vi "F.L.Y Stick Controller.vi"   [LabVIEW 2019]
uses:
  <vilib>/Rock Robotics/WPI/Joystick/WPI_JoystickDeviceEnum.ctl
  F.L.Y Stick Controller Global.vi
types:
  T1 = typedef "WPI_JoystickDeviceEnum.ctl" = enum16{"USB 0", "USB 1", "USB 2", "USB 3", "USB 4", "USB 5"}
  T2 = typedef "WPI_JoystickDevRef.ctl" = cluster{"Device":T1}
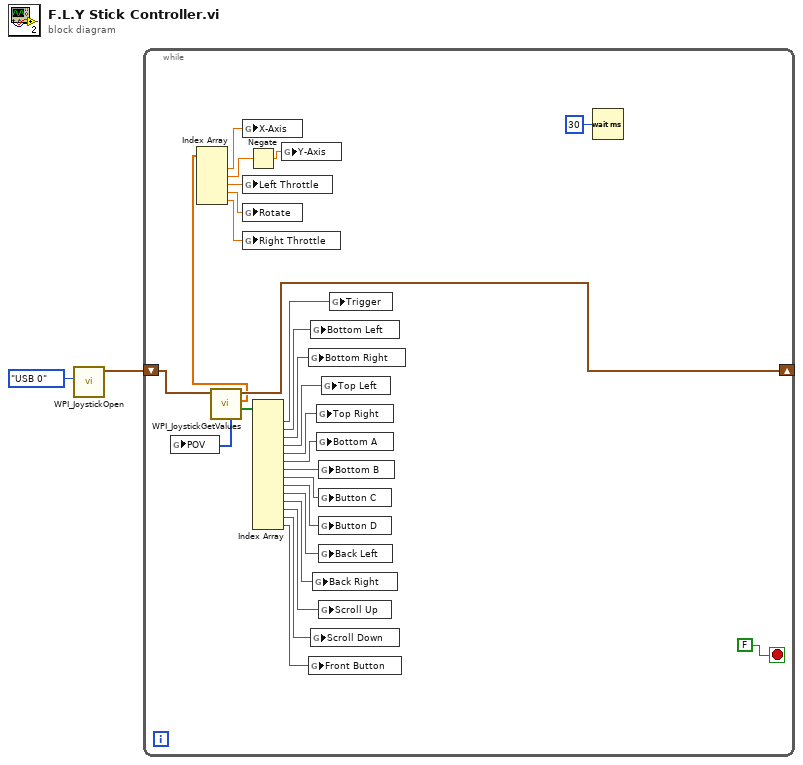
[diagram p0: block diagram]
diagram:
  n1 = call <vilib>:"WPI_JoystickOpen.vi"("JoystickDevice"=WPI_JoystickDeviceEnum."USB 0") -> ("JoystickDevRef"=w2:T2)  [unwired: 10 in]
  n2 = while {
    shift-right: [w27] -> _
    shift-left: w2 -> [w28]
    stop <- FALSE stop-if-true
    n3 = call <vilib>:"WPI_JoystickGetValues.vi"("JoystickDevRef"=w28) -> ("Buttons"=w26:bool[], "Axes"=w11:dbl[], "JoystickDevRef"=w27:T2, "POVs"=w6:i16[])  [unwired: 6 in, 1 out]
    n4 = global write "F.L.Y Stick Controller Global.vi" "POV"(w6) -> ()
    n5 = Index Array(array=w11) -> (element #1=w10:dbl, element #2=w3:dbl, element #3=w9:dbl, element #4=w8:dbl, element #5=w7:dbl)  [unwired: 5 in]
    n6 = global write "F.L.Y Stick Controller Global.vi" "X-Axis"(w10) -> ()
    n7 = global write "F.L.Y Stick Controller Global.vi" "Left Throttle"(w9) -> ()
    n8 = global write "F.L.Y Stick Controller Global.vi" "Rotate"(w8) -> ()
    n9 = global write "F.L.Y Stick Controller Global.vi" "Right Throttle"(w7) -> ()
    n10 = Negate(x=w3) -> (-x=w4:dbl)
    n11 = Index Array(array=w26) -> (element #1=w25:bool, element #2=w24:bool, element #3=w23:bool, element #4=w22:bool, element #5=w21:bool, element #6=w20:bool, element #7=w19:bool, element #8=w18:bool, element #9=w17:bool, element #10=w16:bool, element #11=w15:bool, element #12=w14:bool, element #13=w13:bool, element #14=w12:bool)  [unwired: 14 in]
    n12 = global write "F.L.Y Stick Controller Global.vi" "Y-Axis"(w4) -> ()
    n13 = global write "F.L.Y Stick Controller Global.vi" "Bottom Right"(w23) -> ()
    n14 = global write "F.L.Y Stick Controller Global.vi" "Front Button"(w12) -> ()
    n15 = global write "F.L.Y Stick Controller Global.vi" "Bottom Left"(w24) -> ()
    n16 = global write "F.L.Y Stick Controller Global.vi" "Scroll Down"(w13) -> ()
    n17 = global write "F.L.Y Stick Controller Global.vi" "Back Right"(w15) -> ()
    n18 = global write "F.L.Y Stick Controller Global.vi" "Top Right"(w21) -> ()
    n19 = global write "F.L.Y Stick Controller Global.vi" "Bottom A"(w20) -> ()
    n20 = global write "F.L.Y Stick Controller Global.vi" "Bottom B"(w19) -> ()
    n21 = global write "F.L.Y Stick Controller Global.vi" "Button C"(w18) -> ()
    n22 = global write "F.L.Y Stick Controller Global.vi" "Button D"(w17) -> ()
    n23 = global write "F.L.Y Stick Controller Global.vi" "Back Left"(w16) -> ()
    n24 = global write "F.L.Y Stick Controller Global.vi" "Scroll Up"(w14) -> ()
    n25 = global write "F.L.Y Stick Controller Global.vi" "Top Left"(w22) -> ()
    n26 = global write "F.L.Y Stick Controller Global.vi" "Trigger"(w25) -> ()
    n27 = Wait (ms)(milliseconds to wait=u32 30) -> ()  [unwired: 1 out]
  }
